vi "Test Launch.vi"   [LabVIEW 2014]
uses:
  Instr Actor/Instr Actor.lvclass
  <vilib>/ActorFramework/Actor/Actor.lvclass
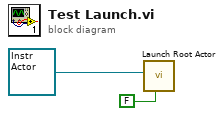
[diagram p0: block diagram]
diagram:
  n1 = call <vilib>:"Launch Root Actor.vi"("Open Actor Core front panel? (F)"=FALSE, "Actor"=refnum<class "Instr Actor.lvclass"> refnum ("Instrument Lib:Instr")) -> ()  [unwired: 8 in, 2 out]
